vi "lesson 2_2.vi"() -> ()   [LabVIEW 2013]
uses:
  <vilib>/sound2/lvsound2.llb/Sampling Mode.ctl
  <vilib>/sound2/lvsound2.llb/Sound Data Format.ctl
  <vilib>/sound2/lvsound2.llb/Sound Input Read (DBL).vi
panel:
  out "Waveform Graph":waveform(dbl)[](graph)
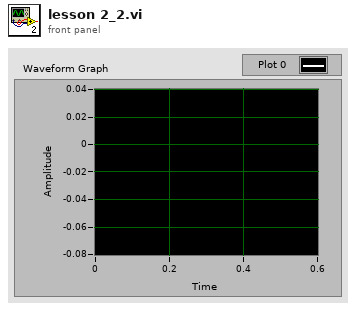
[diagram p1: front panel]
types:
  T1 = typedef "Sound Data Format.ctl" = cluster{"sample rate (S/s)":dbl, "number of channels":i32, "bits per sample":i32}
  T2 = typedef "Sampling Mode.ctl" = i32
  T3 = typedef "Sound Input Task ID.ctl" = u32
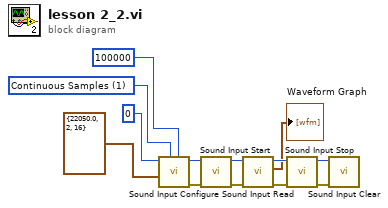
[diagram p0: block diagram]
diagram:
  w4 = T2 1 items=["Finite Samples", "Continuous Samples"] ("sample mode")
  n1 = call <vilib>:"Sound Input Configure.vi"("number of samples/ch"=100000, "sample mode"=w4, "sound format"=T1 {"sample rate (S/s)"=22050.0, "number of channels"=2, "bits per sample"=16}, "device ID"=u32 0) -> ("error out"=w13:errorcluster, "task ID"=w12:T3)  [unwired: 6 in]
  n2 = call <vilib>:"Sound Input Start.vi"("error in (no error)"=w13, "task ID"=w12) -> ("error out"=w11:errorcluster, "task ID out"=w10:T3)  [unwired: 8 in]
  n3 = call-poly <vilib>:"Sound Input Read.vi"("error in (no error)"=w11, "task ID"=w10) -> ("error out"=w9:errorcluster, "data"=→"Waveform Graph":waveform(dbl)[], "task ID out"=w8:T3)  [unwired: 7 in]
  n4 = call <vilib>:"Sound Input Stop.vi"("error in (no error)"=w9, "task ID"=w8) -> ("error out"=w7:errorcluster, "task ID out"=w6:T3)  [unwired: 8 in]
  n5 = call <vilib>:"Sound Input Clear.vi"("error in (no error)"=w7, "task ID"=w6) -> ()  [unwired: 9 in, 1 out]
